vi "Init.vi"(8 "error in (no error)":errorcluster, 11 "USD Actor in":refnum<class "USD Actor.lvclass">) -> (0 "error out":errorcluster, 3 "USD Actor out":refnum<class "USD Actor.lvclass">)   [LabVIEW 2019, in "USD Actor.lvlib" / "USD Actor.lvclass"]
uses:
  USD Actor.lvclass
  USD Actor.lvclass/USD Actor.ctl
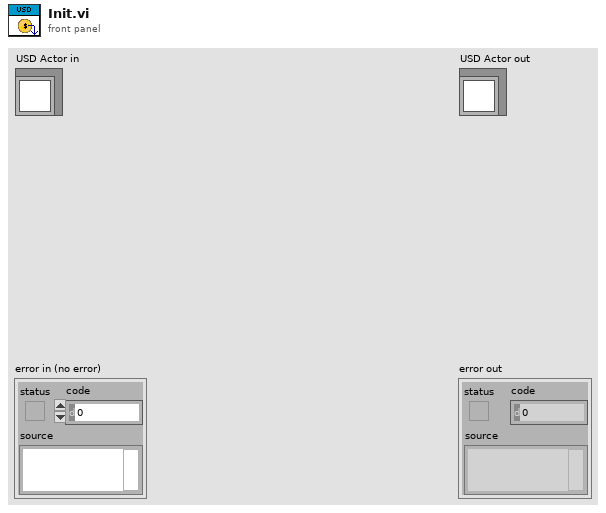
[diagram p1: front panel]
types:
  T1 = cluster{"MONEDAS[0]":string, "MONEDAS[1]":string, "MONEDAS[2]":string, "MONEDAS[3]":string, "MONEDAS[4]":string, "MONEDAS[5]":string, "MONEDAS[6]":string, "MONEDAS[7]":string, "MONEDAS[8]":string}
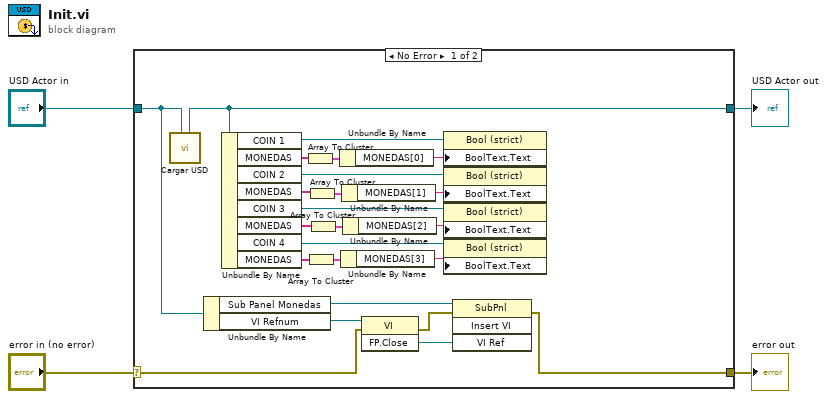
[diagram p0: block diagram]
diagram:
  n1 = case shown="No Error" "error in (no error)" {
    selector: "error in (no error)" -> [w24 w30]
    tunnel: [w23 w30] -> w3
    tunnel: [w5 w29] -> w1
    tunnel: "USD Actor in" -> [w6 w29]
    frame No Error {
      n2 = call "Cargar USD.vi"("USD Actor.lvlib:USD Actor.lvclass"=w6) -> ("USD Actor.lvlib:USD Actor.lvclass 2"=w5:refnum<class "USD Actor.lvclass">)  [unwired: 10 in]
      n3 = Unbundle By Name(w6) -> ("Sub Panel Monedas"=w28:refnum<vi>, "VI Refnum"=w27:refnum<vi>)
      n4 = Unbundle By Name(w5) -> ("COIN 1"=w14:refnum<vi>, "MONEDAS"=w15:string[], "COIN 2"=w12:refnum<vi>, "MONEDAS"=w17:string[], "COIN 3"=w7:refnum<vi>, "MONEDAS"=w19:string[], "COIN 4"=w9:refnum<vi>, "MONEDAS"=w21:string[])
      n5 = Array To Cluster(array=w15) -> (cluster=w16:T1)
      n6 = Array To Cluster(array=w21) -> (cluster=w22:T1)
      n7 = Array To Cluster(array=w17) -> (cluster=w18:T1)
      n8 = Array To Cluster(array=w19) -> (cluster=w20:T1)
      n9 = Unbundle By Name(w16) -> ("MONEDAS[0]"=w13:string)
      n10 = Unbundle By Name(w22) -> ("MONEDAS[3]"=w8:string)
      n11 = Unbundle By Name(w18) -> ("MONEDAS[1]"=w11:string)
      n12 = Unbundle By Name(w20) -> ("MONEDAS[2]"=w10:string)
      n13 = invoke class="VI" method="FP.Close"(reference=w27, error in=w24) -> (reference out=w26:refnum<vi>, error out=w25:errorcluster)  [unwired: 1 in, 1 out]
      n14 = property class="Bool (strict)"(reference=w14, "BoolText.Text"=w13) -> ()  [unwired: 1 in, 2 out]
      n15 = property class="Bool (strict)"(reference=w12, "BoolText.Text"=w11) -> ()  [unwired: 1 in, 2 out]
      n16 = property class="Bool (strict)"(reference=w7, "BoolText.Text"=w10) -> ()  [unwired: 1 in, 2 out]
      n17 = property class="Bool (strict)"(reference=w9, "BoolText.Text"=w8) -> ()  [unwired: 1 in, 2 out]
      n18 = invoke class="SubPnl" method="Insert VI"(reference=w28, error in=w25, "VI Ref"=w26) -> (error out=w23:errorcluster)  [unwired: 1 in, 3 out]
    }
    frame Error {
    }
  }
  "error out" <- w3
  "USD Actor out" <- w1
